vi "lsl create continuous resolver byprop.vi"(8 "error in (no error)":errorcluster, 9 "forget_after":dbl, 10 "value":string, 11 "prop":string) -> (0 "error out":errorcluster, 3 "function return":u32)   [LabVIEW 2018, in "liblsl-LabVIEW.lvlib"]
doc: "extern LIBLSL_C_API lsl_continuous_resolver lsl_create_continuous_resolver_byprop(const char *prop, const char *value, double forget_after);"
uses:
  <userlib>/liblsl-LabVIEW/liblsl-LabVIEW.lvlib
  <userlib>/liblsl-LabVIEW/liblsl64.dll
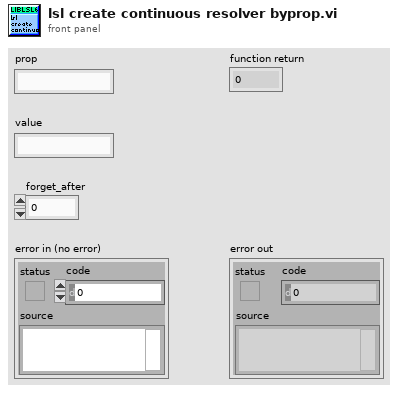
[diagram p1: front panel]
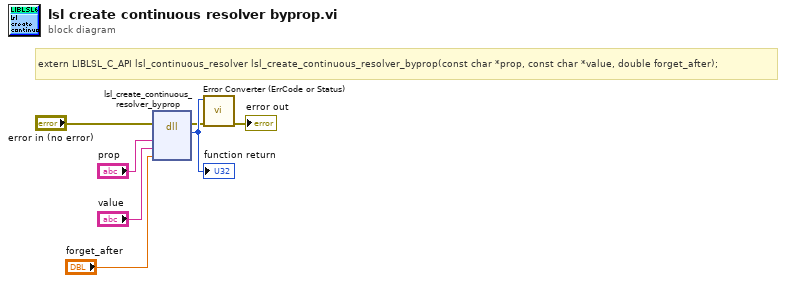
[diagram p0: block diagram]
diagram:
  # "extern LIBLSL_C_API lsl_continuous_resolver lsl_create_continuous_resolver_byprop(const char *prop, const char *value, double forget_after);"
  n1 = dll-call lib="C:/Program Files/National Instruments/LabVIEW 2018/user.lib/liblsl-LabVIEW/liblsl64.*" fn="lsl_create_continuous_resolver_byprop"(error in="error in (no error)", "prop"="prop", "value"="value", "forget_after"="forget_after") -> (error out=w2:errorcluster, w7:u32)  [unwired: 5 in, 1 out]
  "function return" <- w7
  n2 = call <userlib>:"Error Converter (ErrCode or Status).vi"("error in (no error)"=w2, "error code"=w7) -> ("error out"=→"error out":errorcluster)  [unwired: 9 in]
